vi "Register Schema From File.vi"(8 "error in":errorcluster, 11 "file (use dialog)":path) -> (0 "error out":errorcluster, 3 "schema id":string)   [LabVIEW 2024]
uses:
  <vilib>/Plug-In SDKs/Clients/Metadata Store V1/Metadata Store Client.lvlibp/API/Metadata Store V1/Register Schema (String).vi
  <vilib>/Plug-In SDKs/Clients/Metadata Store V1/Metadata Store Client.lvlibp
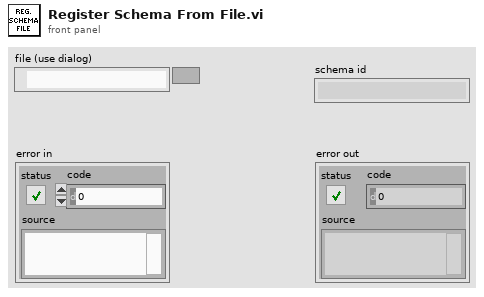
[diagram p1: front panel]
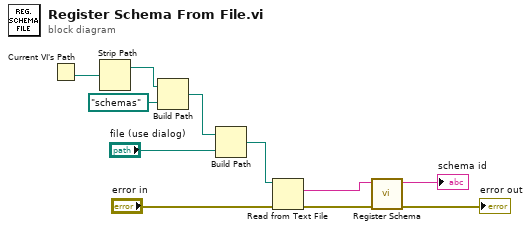
[diagram p0: block diagram]
diagram:
  n1 = Current VI's Path() -> (path=w11:path)
  n2 = Strip Path(path=w11) -> (stripped path=w3:path)  [unwired: 1 out]
  n3 = Build Path(base path=w3, name or relative path=path "schemas") -> (appended path=w2:path)
  n4 = Build Path(base path=w2, name or relative path="file (use dialog)") -> (appended path=w6:path)
  n5 = Read from Text File(file (use dialog)=w6, error in="error in") -> (text=w7:string, error out=w8:errorcluster)  [unwired: 2 in, 2 out]
  n6 = call-poly <vilib>:"Register Schema.vi"("error in"=w8, "schema"=w7) -> ("error out"=→"error out":errorcluster, "schema id"=→"schema id":string)  [unwired: 8 in]
